vi "Resample Blend.vi"(6 "Length":dbl=1.0, 8 "Speeds in":T1={"maxV (fps)"=20.0, "Accel Limit (fps^2)"=20.0, "Initial V (fps)"=0.0, "Sample Period (s)"=0.02, "Jerk Limit (fps^3)"=0.0, "Distances"=[]}, 9 "Initial Point":cluster{"x":dbl, "y":dbl, "th":dbl}={"x"=1.0, "y"=2.0, "th"=30.0}, 10 "Point Arrays":cluster{dbl[], dbl[], dbl[]}, 11 "Initial Acceleration":dbl format="%#_13g") -> (0 "Speeds out":T1={"maxV (fps)"=20.0, "Accel Limit (fps^2)"=20.0, "Initial V (fps)"=0.0, "Sample Period (s)"=0.02, "Jerk Limit (fps^3)"=0.0, "Distances"=[]}, 1 "Vel Points":cluster{dbl, dbl}[](array[cluster]), 2 "Points":cluster{dbl, dbl}[](array[cluster]), 3 "Indices":cluster{"Accel Index":i32, "Decel Index":i32}, 5 "Final Acceleration":dbl)   [LabVIEW 2025]
uses:
  Types/Speeds.ctl
panel:
  out "Array":dbl[](array[numeric])
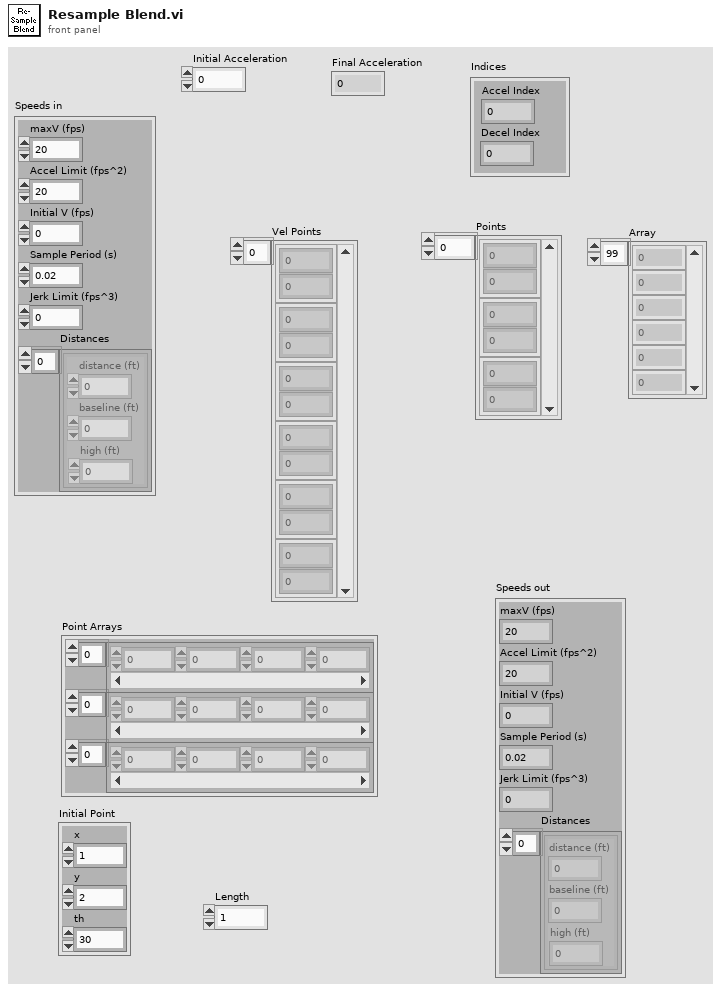
[diagram p1: front panel]
types:
  T1 = typedef "Speeds.ctl" = cluster{"maxV (fps)":dbl, "Accel Limit (fps^2)":dbl, "Initial V (fps)":dbl, "Sample Period (s)":dbl, "Jerk Limit (fps^3)":dbl, "Distances":cluster{"distance (ft)":dbl, "baseline (ft)":dbl, "high (ft)":dbl}[]}
  T2 = cluster{"distance (ft)":dbl, "baseline (ft)":dbl, "high (ft)":dbl}[]
  T3 = cluster{"Initial Acceleration":dbl, "Initial V (fps)":dbl}
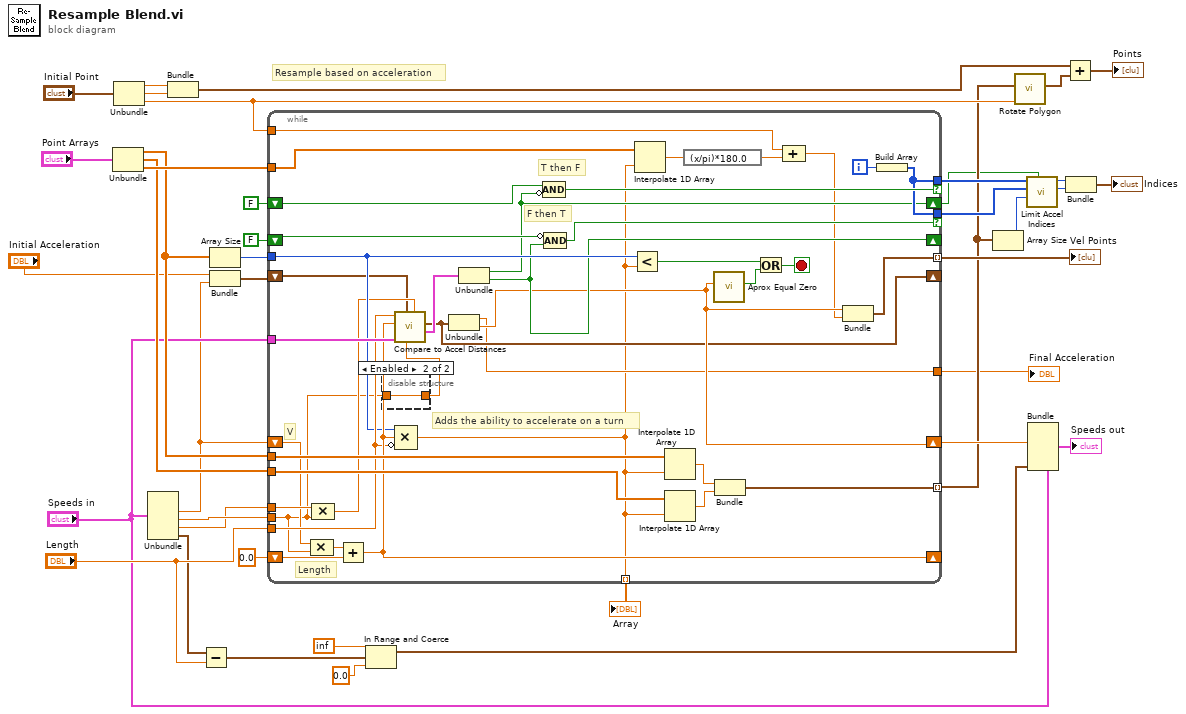
[diagram p0: block diagram]
diagram:
  # "Resample based on acceleration"
  n1 = Unbundle("Point Arrays") -> (w34:dbl[], w35:dbl[], w36:dbl[])
  n2 = Unbundle("Initial Point") -> ("x"=w31:dbl, "y"=w32:dbl, "th"=w30:dbl)
  n3 = Unbundle("Speeds in") -> ("Initial V (fps)"=w6:dbl, "Sample Period (s)"=w40:dbl, "Jerk Limit (fps^3)"=w9:dbl, "Distances"=w3:T2)  [unwired: 2 out]
  n4 = Bundle("x"=w31, "y"=w32) -> (w29:cluster{"x":dbl, "y":dbl})  [unwired: 1 in]
  n5 = Subtract(x=w3, y="Length") -> (x-y=w25:T2)
  n6 = Array Size(array=w34) -> (size(s)=w23:i32)
  n7 = Bundle("Initial Acceleration"="Initial Acceleration", "Initial V (fps)"=w6) -> (w8:T3)  [unwired: 1 in]
  n8 = while {
    tunnel: w34 -> [w79]
    tunnel: w35 -> [w78]
    tunnel: [w75] -> w16 mode=indexing
    tunnel: w40 -> [w45]
    shift-right: [w49] -> w39
    shift-left: w6 -> [w51]
    tunnel: w9 -> [w74]
    tunnel: w23 -> [w56]
    tunnel: w36 -> [w73]
    tunnel: w30 -> [w71]
    shift-right: [w53] -> w4
    shift-left: FALSE -> [w70]
    tunnel: [w59] -> w20 if=w69
    tunnel: "Length" -> [w57]
    tunnel: "Speeds in" -> [w68]
    shift-right: [w52] -> _
    shift-left: FALSE -> [w67]
    tunnel: [w59] -> w19 if=w66
    tunnel: [w63] -> w21 mode=indexing
    shift-right: [w58] -> _
    shift-left: 0.0 -> [w62]
    shift-right: [w48] -> _
    shift-left: w8 -> [w47]
    tunnel: [w44] -> w5
    tunnel: [w41] -> w1 mode=indexing
    i -> [w60]
    stop <- w64 stop-if-true
    # "F then T"
    # "T then F"
    # "Adds the ability to accelerate on a turn"
    # "Length"
    # "V"
    n9 = Compound Arithmetic op=MULTIPLY(w51, w45) -> (w61:dbl)
    n10 = Compound Arithmetic op=MULTIPLY(w74, w45) -> (w50:dbl)
    n11 = Add(x=w61, y=w62) -> (x+y=w58:dbl)
    n12 = disable-structure shown="Enabled" {
      disable-tunnel: [_ w80] -> w46
      disable-tunnel: w45 -> [_ w80]
      frame Disabled {
      }
      frame Enabled {
      }
    }
    n13 = call "Compare to Accel Distances.vi"("dA"=w50, "Sample Period (s)"=w46, "Values"=w47, "Speeds in"=w68, "Current  Length"=w58, "Total Segment Length"=w57) -> ("Ends"=w54:cluster{"Accel End":bool, "Decel End":bool}, "Values out"=w48:cluster{"accel":dbl, "velocity":dbl})  [unwired: 2 in, 2 out]
    n14 = Compound Arithmetic op=MULTIPLY(w56, w58, invert w57) -> (w41:dbl)
    n15 = Unbundle(w48) -> ("accel"=w44:dbl, "velocity"=w49:dbl)
    n16 = Unbundle(w54) -> ("Accel End"=w53:bool, "Decel End"=w52:bool)
    n17 = Compound Arithmetic op=AND(w70, invert w53) -> (w69:bool)
    n18 = Compound Arithmetic op=AND(invert w67, w52) -> (w66:bool)
    n19 = Less?(x=w56, y=w41) -> (x < y?=w65:bool)
    n20 = Interpolate 1D Array(1:w41, 2:w73) -> (0:w72:dbl)
    n21 = Interpolate 1D Array(1:w41, 2:w79) -> (0:w77:dbl)
    n22 = Interpolate 1D Array(1:w41, 2:w78) -> (0:w76:dbl)
    n23 = expression code="(x/pi)*180.0" ("radians to degrees")(w72) -> (w43:dbl)
    n24 = call "Aprox Equal Zero.vi"("x"=w49) -> ("Boolean"=w55:bool)  [unwired: 10 in]
    n25 = Bundle(w77, w76) -> (w75:cluster{dbl, dbl})  [unwired: 1 in]
    n26 = Or(x=w65, y=w55) -> (x .or. y?=w64:bool)
    n27 = Compound Arithmetic op=ADD(w71, w43) -> (w42:dbl)
    n28 = Bundle("velocity"=w49, w42) -> (w63:cluster{"velocity":dbl, dbl})  [unwired: 1 in]
    n29 = Build Array(w60) -> (w59:i32[])
  }
  "Vel Points" <- w21
  "Final Acceleration" <- w5
  "Array" <- w1
  n30 = In Range and Coerce(upper limit=inf, x=w25, lower limit=0.0) -> (coerced(x)=w2:T2)  [unwired: 1 out]
  n31 = Array Size(array=w16) -> (size(s)=w15:i32)
  n32 = call "Rotate Polygon.vi"("Angle"=w30, "polygon 2"=w16) -> ("polygon"=w28:cluster{dbl, dbl}[])  [unwired: 9 in]
  n33 = call "Limit Accel Indices.vi"("Last Accel"=w4, "Size"=w15, "Decel"=w19, "Accel"=w20) -> ("Decel Index"=w17:i32, "Accel Index"=w18:i32)  [unwired: 6 in]
  n34 = Bundle(cluster="Speeds in", "Initial V (fps)"=w39, "Distances"=w2) -> (→"Speeds out":T1)  [unwired: 4 in]
  n35 = Add(x=w29, y=w28) -> (x+y=→"Points":cluster{dbl, dbl}[])
  n36 = Bundle("Accel Index"=w18, "Decel Index"=w17) -> (→"Indices":cluster{"Accel Index":i32, "Decel Index":i32})  [unwired: 1 in]
